vi "decode access token response.vi"(8 "error in (no error)":errorcluster, 9 "Response":string, 10 "Header":string, 11 "Oauth2 in":refnum<class "Oauth2.lvclass">) -> (0 "error out":errorcluster, 1 "Token Type":string, 2 "Access Token":string, 3 "Oauth2":refnum<class "Oauth2.lvclass">, 5 "Scope":string)   [LabVIEW 2013, in "Oauth2.lvclass"]
uses:
  Oauth2.lvclass
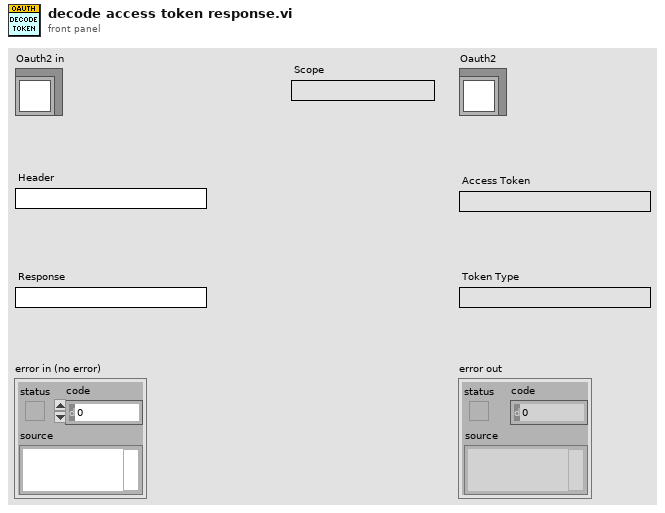
[diagram p1: front panel]
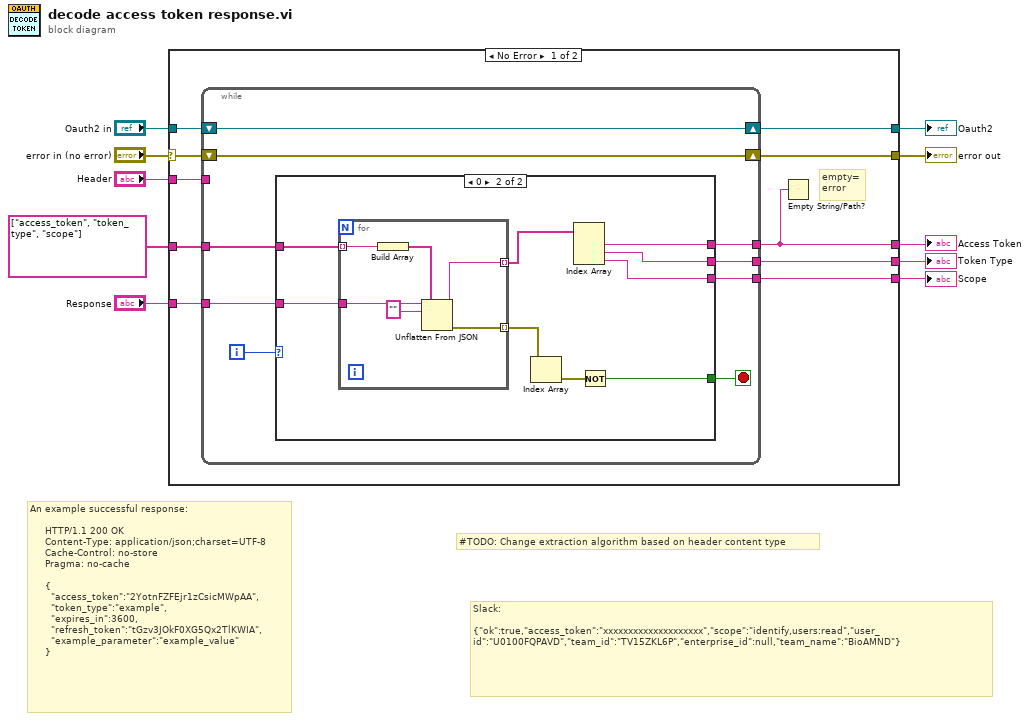
[diagram p0: block diagram]
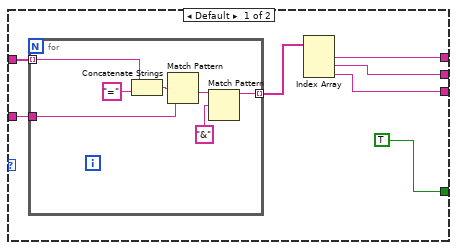
[diagram p2: hidden frame]
diagram:
  # "Slack:\n\n{\"ok\":true,\"access_token\":\"xxxxxxxxxxxxxxxxxxxx\",\"scope\":\"identify,users:read\",\"user_id\":\"U0100FQPAVD\",\"team_id\":\"TV15ZKL6P\",\"enterprise_id\":null,\"team_name\":\"BioAMND\"}"
  # "#TODO: Change extraction algorithm based on header content type"
  # "An example successful response:\n\n     HTTP/1.1 200 OK\n     Content-Type: application/json;charset=UTF-8\n     Cache-Control: no-store\n     Pragma: no-cache\n\n     {\n       \"access_token\":\"2YotnFZFEjr1zCsicMWpAA\",\n       \"token_type\":\"example\",\n       \"expires_in\":3600,\n       \"refresh_token\":\"tGzv3JOkF0XG5Qx2TlKWIA\",\n       \"example_parameter\":\"example_value\"\n     }"
  n1 = case shown="No Error" "error in (no error)" {
    selector: "error in (no error)" -> [w16 w61]
    tunnel: [w17 w61] -> w9
    tunnel: [w18 w60] -> w7
    tunnel: "Oauth2 in" -> [w19 w60]
    tunnel: [w15 w59] -> w6
    tunnel: "Response" -> [w20 w59]
    tunnel: [w14 _] -> w4
    tunnel: [w13 _] -> w3
    tunnel: string[] ["access_token", "token_type", "scope"] -> [w12 _]
    tunnel: "Header" -> [w11 _]
    frame No Error {
      # "empty=\nerror"
      n2 = while {
        tunnel: w20 -> [w29]
        shift-right: [w28] -> w18
        shift-left: w19 -> [w28]
        shift-right: [w27] -> w17
        shift-left: w16 -> [w27]
        tunnel: [w24] -> w15
        tunnel: [w23] -> w14
        tunnel: [w22] -> w13
        tunnel: w12 -> [w21]
        tunnel: w11 -> [_]
        i -> [w25]
        stop <- w26 stop-if-true
        n3 = case shown="0" w25 {
          tunnel: w29 -> [w35 w52]
          tunnel: [w32 w46] -> w24
          tunnel: [TRUE w47] -> w26
          tunnel: [w31 w45] -> w23
          tunnel: [w30 w44] -> w22
          tunnel: w21 -> [w34 w51]
          frame Default {
            n4 = for {
              tunnel: w35 -> [w43]
              tunnel: [w40] -> w33 mode=indexing
              tunnel: w34 -> [w37] mode=indexing
              n5 = Concatenate Strings(w37, "=" ("regular expression")) -> (w38:string)
              n6 = Match Pattern(string=w43, regular expression=w38) -> (after substring=w42:string)  [unwired: 1 in, 3 out]
              n7 = Match Pattern(string=w42, regular expression="&") -> (before substring=w40:string)  [unwired: 1 in, 3 out]
            }
            n8 = Index Array(array=w33) -> (element #1=w32:string, element #2=w31:string, element #3=w30:string)  [unwired: 3 in]
          }
          frame 0 {
            n9 = for {
              tunnel: [w53] -> w50 mode=indexing
              tunnel: w52 -> [w58]
              tunnel: [w57] -> w49 mode=indexing
              tunnel: w51 -> [w55] mode=indexing
              n10 = Build Array(w55) -> (w54:string[])
              n11 = Unflatten From JSON(path=w54, JSON string=w58, type and defaults="") -> (value=w53:string, error out=w57:errorcluster)  [unwired: 4 in]
            }
            n12 = Index Array(array=w49) -> (element=w48:errorcluster)  [unwired: 1 in]
            n13 = Index Array(array=w50) -> (element #1=w46:string, element #2=w45:string, element #3=w44:string)  [unwired: 3 in]
            n14 = Not(x=w48) -> (.not. x?=w47:bool)
          }
        }
      }
      n15 = Empty String/Path?(string/path=w15) -> ()  [unwired: 1 out]
    }
    frame Error {
    }
  }
  "error out" <- w9
  "Oauth2" <- w7
  "Access Token" <- w6
  "Scope" <- w3
  "Token Type" <- w4
